vi "Message to RT.vi"(8 "error in (no error)":errorcluster, 9 "Message Data":variant, 10 "Message":string, 11 "Connected(T)":bool=TRUE) -> (0 "error out":errorcluster)   [LabVIEW 2015, in "Tool Interface.lvlib"]
uses:
  Tool Typedefs/Message Cluster.ctl
  Tool Interface.lvlib
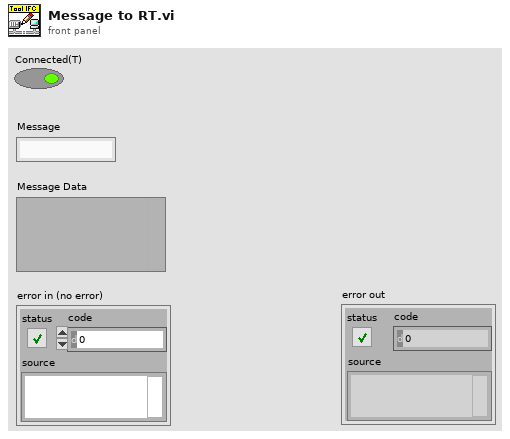
[diagram p1: front panel]
types:
  T1 = typedef "Message Cluster.ctl" = cluster{"Message":string, "Message Data":variant}
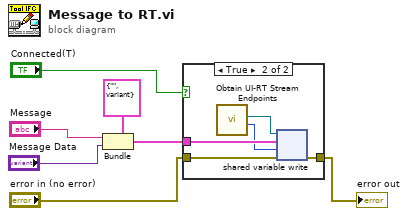
[diagram p0: block diagram]
diagram:
  n1 = Bundle(cluster=T1 {"Message"="", "Message Data"=variant} ("Message Cluster"), "Message"="Message", "Message Data"="Message Data") -> (w4:T1)
  n2 = case shown="True" "Connected(T)" {
    tunnel: "error in (no error)" -> [w8 w13]
    tunnel: [w8 w12] -> w2
    tunnel: w4 -> [_ w10]
    frame False {
    }
    frame True {
      n3 = call "Obtain UI-RT Stream Endpoints.vi"() -> ("Connect Timeout(ms)"=w9:i32, "UI Command Stream"=w11:refnum<k21>)  [unwired: 9 in, 1 out]
      n4 = shared-variable-write(w11, w13, w10, w9) -> (w12:errorcluster)  [unwired: 2 out]
    }
  }
  "error out" <- w2
